vi "Single_Pulse_Debugger.vi"() -> ()   [LabVIEW 2021]
uses:
  Drivers/Arduino_Pulse_Generator/Configurate/Channel_Pulse_Stream.ctl
  Addons/Prepare_Pulse_Sequence/Pulse_Sequence_Global.vi
panel:
  in  "sending step":T1(ring)=enum."initialize"
  in  "Arduino VISA":refnum<visa-resource-name>
  out "pulse seq changed (?)":bool=TRUE
  out "Init outp register 2 (8-13)":bool[](array[boolean])
  out "Init outp register 1 (2-7)":bool[](array[boolean])
  out "Pulse sequence":T2[](array[typedef]) {"channel" min=2 max=13 step=1}
  in  "Run sequence":bool
  in  "Close":bool
  in  "Define pulse sequence":bool
  in  "Define initial states":bool
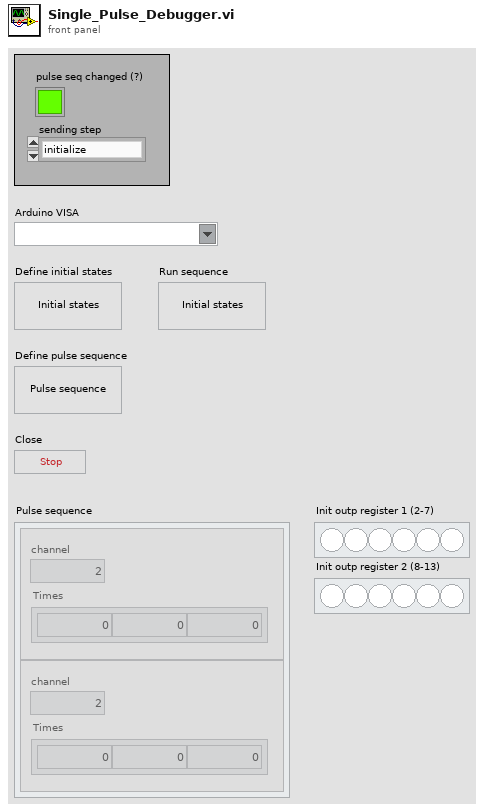
[diagram p1: front panel]
types:
  T1 = enum16{"close", "run", "set pulse", "set initial", "initialize"}
  T2 = typedef "Channel_Pulse_Stream.ctl" = cluster{"Times":dbl[], "channel":u8}
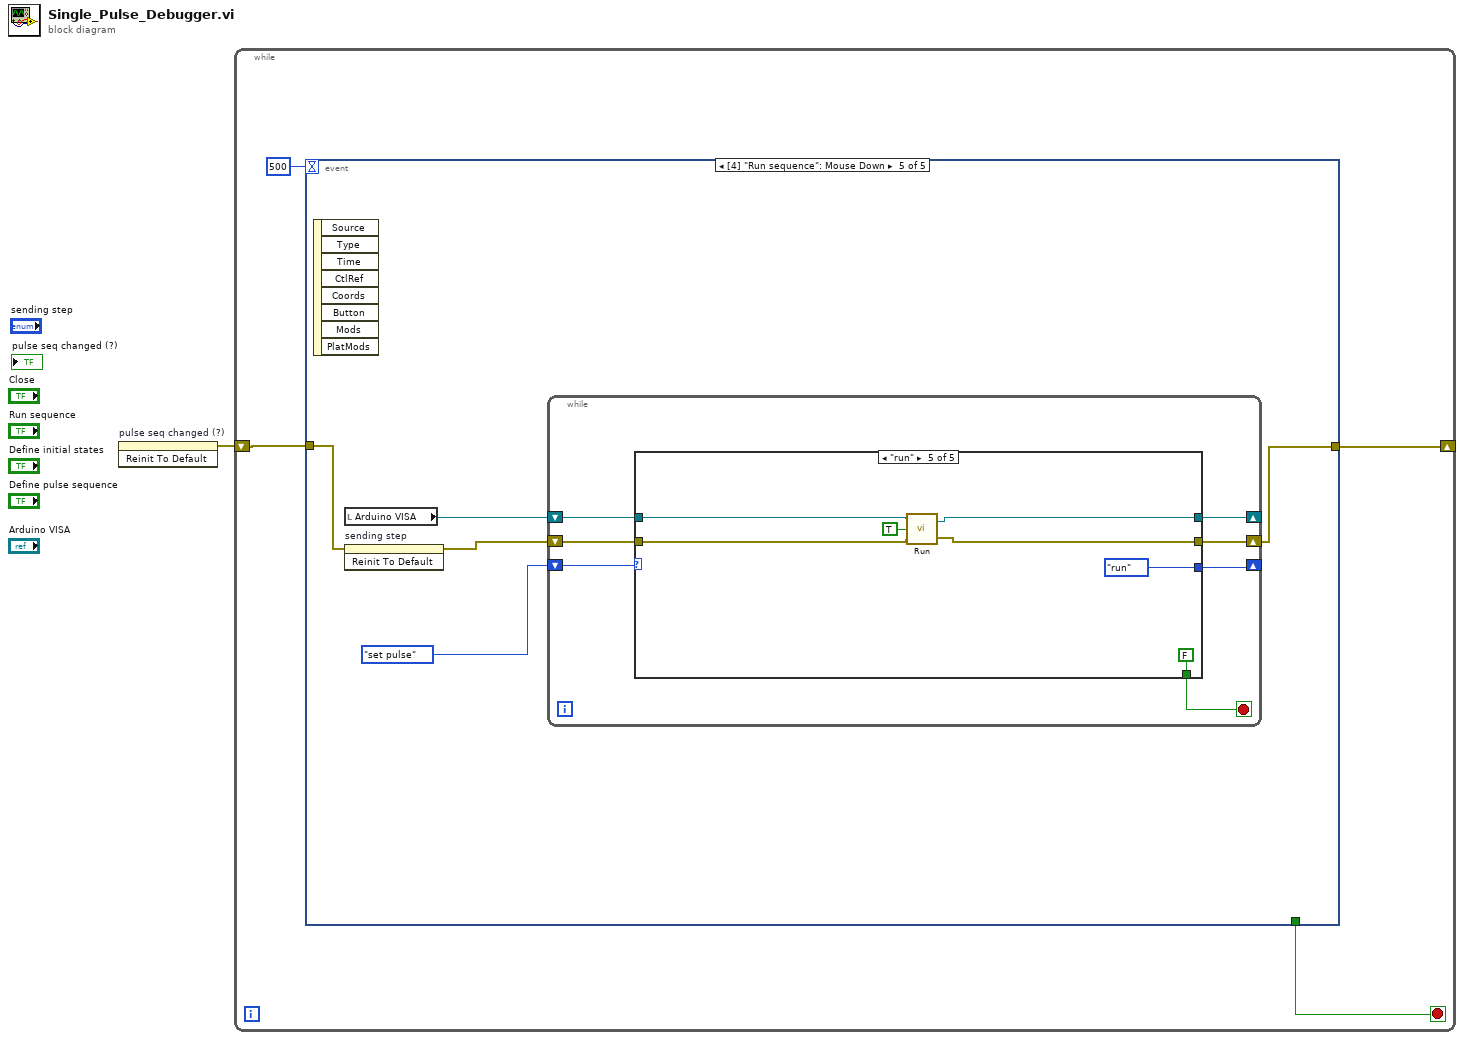
[diagram p0: block diagram]
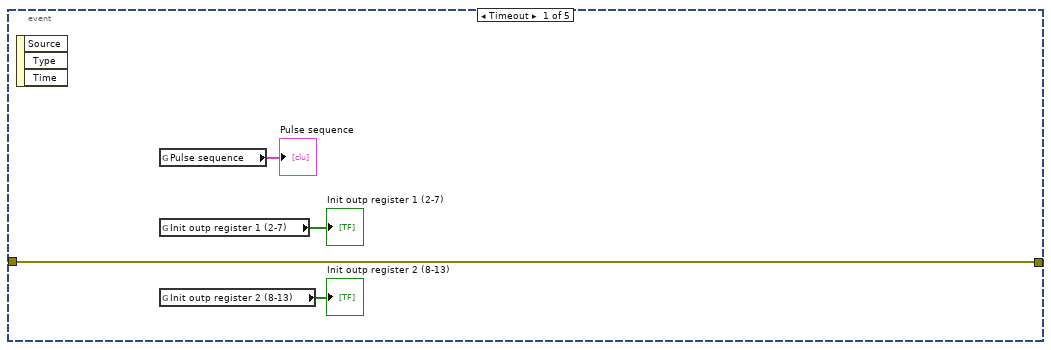
[diagram p2: hidden frame]
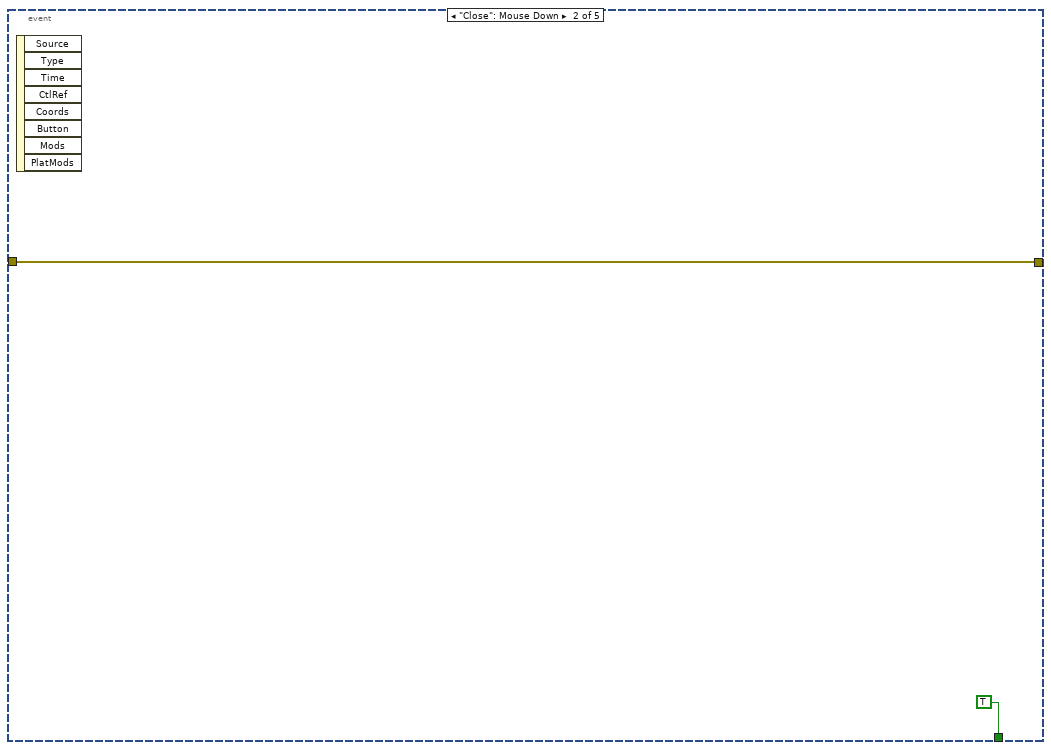
[diagram p3: hidden frame]
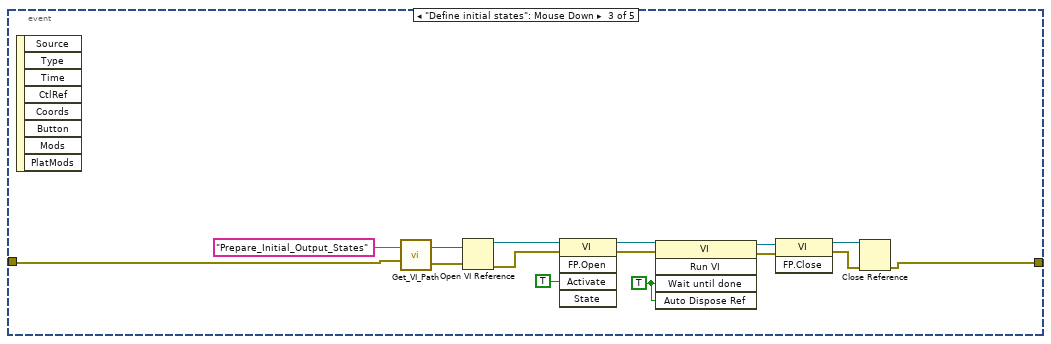
[diagram p4: hidden frame]
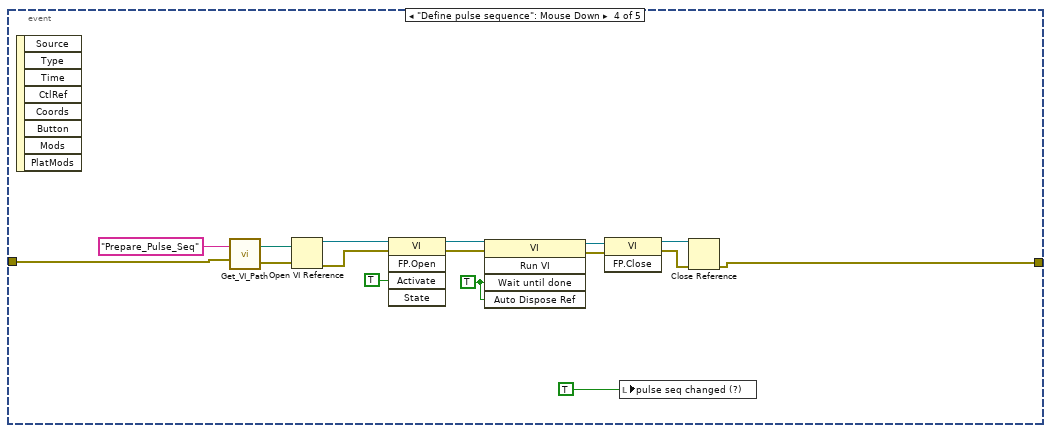
[diagram p5: hidden frame]
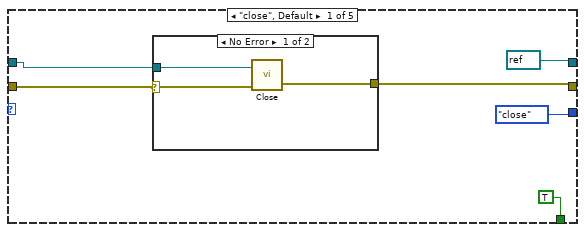
[diagram p6: hidden frame]
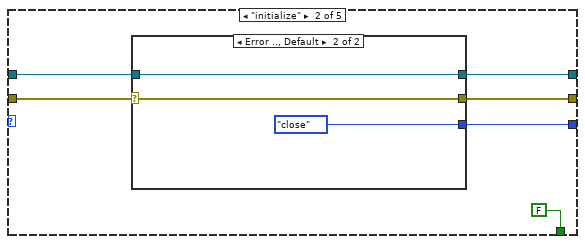
[diagram p8: hidden frame]
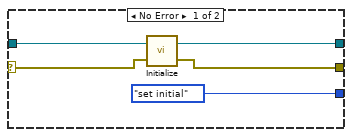
[diagram p9: hidden frame]
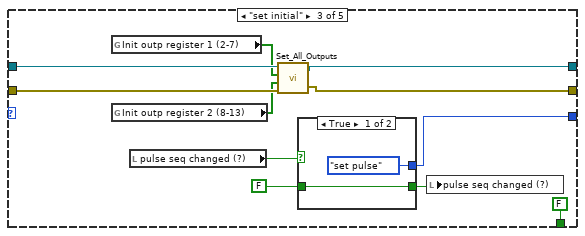
[diagram p10: hidden frame]
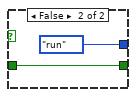
[diagram p11: hidden frame]
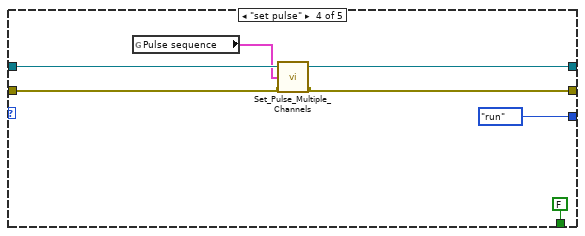
[diagram p12: hidden frame]
diagram:
  n1 = invoke on="pulse seq changed (?)" class="Bool (strict)" method="Reinit To Default"() -> (error out=w1:errorcluster)  [unwired: 3 in, 2 out]
  n2 = while {
    shift-right: [w4] -> _
    shift-left: w1 -> [w5]
    stop <- w2 stop-if-true
    n3 = event shown="[4] \"Run sequence\": Mouse Down" {
      selector: _ -> [_ _ _ _ _]
      dyn-events: _ -> [_ _ _ _ _]
      timeout: 500 -> [_ _ _ _ _]
      tunnel: w5 -> [w6 w10 w13 w29 w46]
      tunnel: [w6 w10 w12 w28 w45] -> w4
      tunnel: [_ TRUE _ _ _] -> w2
      event Timeout {
        n4 = event-data() -> ()  [unwired: 1 in, 3 out]
        n5 = global read "Pulse_Sequence_Global.vi" "Pulse sequence"() -> (→"Pulse sequence":T2[])
        n6 = global read "Pulse_Sequence_Global.vi" "Init outp register 1 (2-7)"() -> (→"Init outp register 1 (2-7)":bool[])
        n7 = global read "Pulse_Sequence_Global.vi" "Init outp register 2 (8-13)"() -> (→"Init outp register 2 (8-13)":bool[])
      }
      event "Close": Mouse Down {
        n8 = event-data() -> ()  [unwired: 1 in, 8 out]
      }
      event "Define initial states": Mouse Down {
        w18 = TRUE ("Wait Until Done")
        n9 = event-data() -> ()  [unwired: 1 in, 8 out]
        n10 = call "Get_VI_Path.vi"("error in"=w13, "VI name (no .vi)"="Prepare_Initial_Output_States") -> ("error out"=w23:errorcluster, "File Path"=w25:path)
        n11 = Open VI Reference(vi path=w25, error in (no error)=w23) -> (vi reference=w24:refnum<vi>, error out=w22:errorcluster)  [unwired: 4 in]
        n12 = invoke class="VI" method="FP.Open"(reference=w24, error in=w22, "Activate"=TRUE ("Activate?")) -> (reference out=w20:refnum<vi>, error out=w19:errorcluster)  [unwired: 2 in, 3 out]
        n13 = invoke class="VI" method="Run VI"(reference=w20, error in=w19, "Wait until done"=w18, "Auto Dispose Ref"=w18) -> (reference out=w17:refnum<vi>, error out=w16:errorcluster)  [unwired: 1 in, 3 out]
        n14 = invoke class="VI" method="FP.Close"(reference=w17, error in=w16) -> (reference out=w15:refnum<vi>, error out=w14:errorcluster)  [unwired: 1 in, 1 out]
        n15 = Close Reference(reference=w15, error in (no error)=w14) -> (error out=w12:errorcluster)
      }
      event "Define pulse sequence": Mouse Down {
        w34 = TRUE ("Wait Until Done")
        n16 = event-data() -> ()  [unwired: 1 in, 8 out]
        n17 = call "Get_VI_Path.vi"("error in"=w29, "VI name (no .vi)"="Prepare_Pulse_Seq") -> ("error out"=w39:errorcluster, "File Path"=w41:path)
        n18 = Open VI Reference(vi path=w41, error in (no error)=w39) -> (vi reference=w40:refnum<vi>, error out=w38:errorcluster)  [unwired: 4 in]
        n19 = invoke class="VI" method="FP.Open"(reference=w40, error in=w38, "Activate"=TRUE ("Activate?")) -> (reference out=w36:refnum<vi>, error out=w35:errorcluster)  [unwired: 2 in, 3 out]
        n20 = invoke class="VI" method="Run VI"(reference=w36, error in=w35, "Wait until done"=w34, "Auto Dispose Ref"=w34) -> (reference out=w33:refnum<vi>, error out=w32:errorcluster)  [unwired: 1 in, 3 out]
        n21 = invoke class="VI" method="FP.Close"(reference=w33, error in=w32) -> (reference out=w31:refnum<vi>, error out=w30:errorcluster)  [unwired: 1 in, 1 out]
        n22 = local write "pulse seq changed (?)"(TRUE ("pulse seq changed (?)")) -> ()
        n23 = Close Reference(reference=w31, error in (no error)=w30) -> (error out=w28:errorcluster)
      }
      event "Run sequence": Mouse Down {
        n24 = event-data() -> ()  [unwired: 1 in, 8 out]
        n25 = local read "Arduino VISA"() -> (w47:refnum<visa-resource-name>)
        n26 = invoke on="sending step" class="Enum (strict)" method="Reinit To Default"(error in=w46) -> (error out=w43:errorcluster)  [unwired: 2 in, 2 out]
        n27 = while {
          shift-right: [w50] -> _
          shift-left: T1."set pulse" ("Enum") -> [w48]
          shift-right: [w52] -> _
          shift-left: w47 -> [w54]
          shift-right: [w51] -> w45
          shift-left: w43 -> [w53]
          stop <- w49 stop-if-true
          n28 = case shown="\"run\"" w48 {
            tunnel: w54 -> [w60 w70 w88 w96 w106]
            tunnel: w53 -> [w56 w66 w86 w99 w104]
            tunnel: [refnum<visa-resource-name> refnum ("Arduino VISA") w69 w87 w97 w105] -> w52
            tunnel: [w59 w68 w85 w98 w103] -> w51
            tunnel: [T1."close" ("Enum") w67 w89 T1."run" ("Enum") T1."run" ("Enum")] -> w50
            tunnel: [TRUE FALSE FALSE FALSE FALSE] -> w49
            frame "close", Default {
              n29 = case shown="No Error" w56 {
                selector: w56 -> [w61 w64]
                tunnel: w60 -> [w63 _]
                tunnel: [w62 w64] -> w59
                frame No Error {
                  n30 = call "Close.vi"("error in"=w61, "VISA arduino in"=w63) -> ("error out"=w62:errorcluster)  [unwired: 1 in]
                }
                frame Error {
                }
              }
            }
            frame "initialize" {
              n31 = case shown="Error .., Default" w66 {
                selector: w66 -> [w71 w76]
                tunnel: w70 -> [w75 w77]
                tunnel: [w74 w77] -> w69
                tunnel: [w73 w76] -> w68
                tunnel: [T1."set initial" ("Enum") T1."close" ("Enum")] -> w67
                frame No Error {
                  n32 = call "Initialize.vi"("error in"=w71, "VISA arduino in"=w75) -> ("error out"=w73:errorcluster, "VISA arduino out"=w74:refnum<visa-resource-name>)
                }
                frame Error, Default {
                }
              }
            }
            frame "set initial" {
              n33 = global read "Pulse_Sequence_Global.vi" "Init outp register 1 (2-7)"() -> (w84:bool[])
              n34 = global read "Pulse_Sequence_Global.vi" "Init outp register 2 (8-13)"() -> (w83:bool[])
              n35 = local read "pulse seq changed (?)"() -> (w82:bool)
              n36 = call "Set_All_Outputs.vi"("error in"=w86, "register 2 (8-13)"=w83, "register 1 (2-7)"=w84, "VISA arduino in"=w88) -> ("error out"=w85:errorcluster, "VISA arduino out"=w87:refnum<visa-resource-name>)
              n37 = case shown="True" w82 {
                tunnel: [T1."set pulse" ("Enum") T1."run" ("Enum")] -> w89
                tunnel: [w90 w92] -> w81
                tunnel: FALSE -> [w90 w92]
                frame True {
                }
                frame False {
                }
              }
              n38 = local write "pulse seq changed (?)"(w81) -> ()
            }
            frame "set pulse" {
              n39 = global read "Pulse_Sequence_Global.vi" "Pulse sequence"() -> (w95:T2[])
              n40 = call "Set_Pulse_Multiple_Channels.vi"("error in"=w99, "Pulses"=w95, "VISA arduino in"=w96) -> ("error out"=w98:errorcluster, "VISA arduino out"=w97:refnum<visa-resource-name>)  [unwired: 1 in]
            }
            frame "run" {
              n41 = call "Run.vi"("error in"=w104, "run?"=TRUE, "VISA arduino in"=w106) -> ("error out"=w103:errorcluster, "VISA arduino out"=w105:refnum<visa-resource-name>)
            }
          }
        }
      }
    }
  }
